vi "GetAttributeViReal64_SA-HD_OB.vi"(8 "error in (no error)":errorcluster {"code" format="%.0x"}, 9 "AttributeID":u32(ring)=1150477 items=["SA_HARMONICDISTORTION_DISPLAYWINDOWY_REFERENCE"=1150477, "SA_HARMONICDISTORTION_DISPLAYWINDOWY_SCALE"=1150479, "SA_HARMONICDISTORTION_FUNDAMENTAL_FREQUENCY"=1150460, "SA_HARMONICDISTORTION_SWEEPCOUPLING_RESOLUTION_BANDWIDTH"=1150464, "SA_HARMONICDISTORTION_SWEEPCOUPLING_SWEEP_TIME"=1150466, "SA_HARMONICDISTORTION_SWEEPCOUPLING_VIDEO_BANDWIDTH"=1150468, "SA_OCCUPIEDBANDWIDTH_DISPLAY_WINDOWY_REFERENCE"=1150309, "SA_OCCUPIEDBANDWIDTH_DISPLAY_WINDOWY_SCALE"=1150312, "SA_OCCUPIEDBANDWIDTH_FREQUENCY_SPAN"=1150299, "SA_OCCUPIEDBANDWIDTH_FREQUENCY_XDB"=1150334, "SA_OCCUPIEDBANDWIDTH_LIMIT_TEST_FREQUENCY"=1150331, "SA_OCCUPIEDBANDWIDTH_MARKER_AMPLITUDE"=1150322, "SA_OCCUPIEDBANDWIDTH_MARKER_FUNCTION_RESULT"=1150327, "SA_OCCUPIEDBANDWIDTH_MARKER_POSITION"=1150328, "SA_OCCUPIEDBANDWIDTH_MARKER_TRACE_POINTS_POSITION"=1150750, "SA_OCCUPIEDBANDWIDTH_PERCENT_POWER"=1150319, "SA_OCCUPIEDBANDWIDTH_SWEEPCOUPLING_RESOLUTION_BANDWIDTH"=1150294, "SA_OCCUPIEDBANDWIDTH_SWEEPCOUPLING_SWEEP_TIME"=1150254, "SA_OCCUPIEDBANDWIDTH_SWEEPCOUPLING_VIDEO_BANDWIDTH"=1150296], 11 "instrument handle":refnum<k15>) -> (0 "error out":errorcluster {"code" format="%.0x"}, 2 "AttributeValue":dbl, 3 "instrument handle out":refnum<k15>)   [LabVIEW 2009, in "Keysight XSAn.lvlib"]
doc: "Gets a Real64 attribute from the instrument driver.\nThe following Attributes are supported:\n\nSA_HARMONICDISTORTION_DISPLAYWINDOWY_REFERENCE\nSA_HARMONICDISTORTION_DISPLAYWINDOWY_SCALE\nSA_HARMONICDISTORTION_FUNDAMENTAL_FREQUENCY\nSA_HARMONICDISTORTION_SWEEPCOUPLING_RESOLUTION_BANDWIDTH\nSA_HARMONICDISTORTION_SWEEPCOUPLING_SWEEP_TIME\nSA_HARMONICDISTORTION_SWEEPCOUPLING_VIDEO_BANDWIDTH\nSA_OCCUPIEDBANDWIDTH_DISPLAY_WINDOWY_REFERENCE\nSA_OCCUPIEDBANDWIDTH_DISPLAY_WINDOWY_SCALE\nSA_OCCUPIEDBANDWIDTH_FREQUENCY_SPAN\nSA_OCCUPIEDBANDWIDTH_FREQUENCY_XDB\nSA_OCCUPIEDBANDWIDTH_LIMIT_TEST_FREQUENCY\nSA_OCCUPIEDBANDWIDTH_MARKER_AMPLITUDE\nSA_OCCUPIEDBANDWIDTH_MARKER_FUNCTION_RESULT\nSA_OCCUPIEDBANDWIDTH_MARKER_POSITION\nSA_OCCUPIEDBANDWIDTH_MARKER_TRACE_POINTS_POSITION\nSA_OCCUPIEDBANDWIDTH_PERCENT_POWER\nSA_OCCUPIEDBANDWIDTH_SWEEPCOUPLING_RESOLUTION_BANDWIDTH\nSA_OCCUPIEDBANDWIDTH_SWEEPCOUPLING_SWEEP_TIME\nSA_OCCUPIEDBANDWIDTH_SWEEPCOUPLING_VIDEO_BANDWIDTH"
uses:
  <instrlib>/Keysight XSAn/Keysight XSAn.lvlib
  AgXSAn.dll
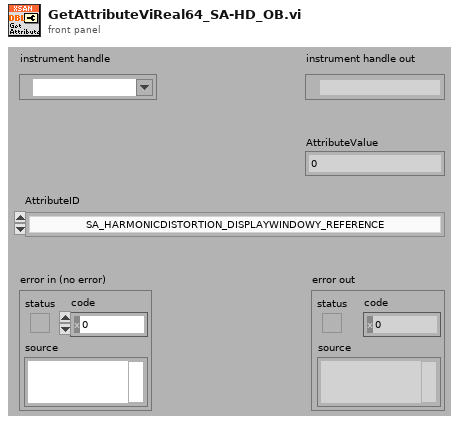
[diagram p1: front panel]
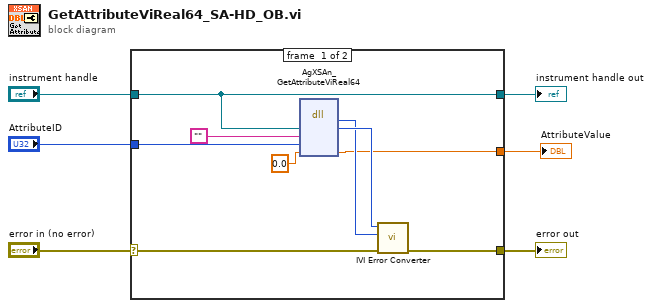
[diagram p0: block diagram]
diagram:
  n1 = case shown="No Error" "error in (no error)" {
    selector: "error in (no error)" -> [w13 w17]
    tunnel: [w12 w17] -> w6
    tunnel: "instrument handle" -> [w8 w16]
    tunnel: "AttributeID" -> [w11 _]
    tunnel: [w9 _] -> w2
    tunnel: [w8 w16] -> w1
    frame #0 {
      n2 = dll-call lib="AgXSAn**.dll" fn="AgXSAn_GetAttributeViReal64"("Vi"=w8, "RepCapIdentifier"="", "AttributeID"=w11, "AttributeValue"=0.0) -> ("return type"=w14:i32, "Vi"=w15:u32, "AttributeValue"=w9:dbl)  [unwired: 5 in, 2 out]
      n3 = call <instrlib>:"IVI Error Converter.vi"("error in (no error)"=w13, "IVI error code (0)"=w14, "instrument handle"=w15) -> ("error out"=w12:errorcluster)  [unwired: 7 in, 1 out]
    }
    frame #1 {
    }
  }
  "error out" <- w6
  "instrument handle out" <- w1
  "AttributeValue" <- w2
